vi "BotSpeak_AnalogOut.vi"(0 "voltage":dbl(knob) scale=0.0..5.0, 2 "Bot Settings":T1, 3 "DAC Channel":u8(slide)=3 scale=0.0..5.0) -> (1 "response":string="169.254.32.85", 4 "Bot Settings":T1)   [LabVIEW 2012]
doc: "Writes the specified \"voltage\" to the specified \"DAC Channel\"."
uses:
  <userlib>/BotSpeak/VIs/Direct/BotSpeak_Control.ctl
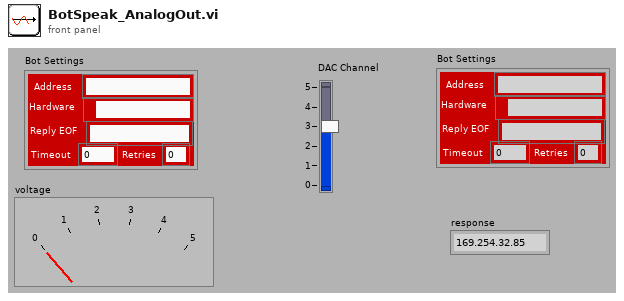
[diagram p1: front panel]
types:
  T1 = typedef "BotSpeak_Control.ctl" = cluster{"Address":string, "Reply EOF":string, "Hardware":path, "Retries":i8, "Timeout":i32}
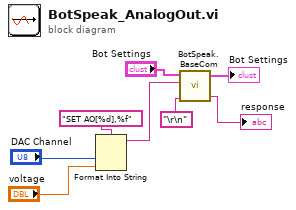
[diagram p0: block diagram]
diagram:
  n1 = Format Into String(format string="SET AO[%d],%f" ("command"), "DAC Channel", "voltage") -> (resulting string=w8:string)  [unwired: 2 in, 1 out]
  n2 = call <userlib>:"BotSpeak.BaseCom.vi"("Termination"="\r\n", "command"=w8, "Bot Settings in"="Bot Settings") -> ("response"=→"response":string, "Bot Settings out"=→"Bot Settings":T1)  [unwired: 2 in]
